vi "Control_HMI.vi"   [LabVIEW 2018]
uses:
  Global/TimerReferences.vi
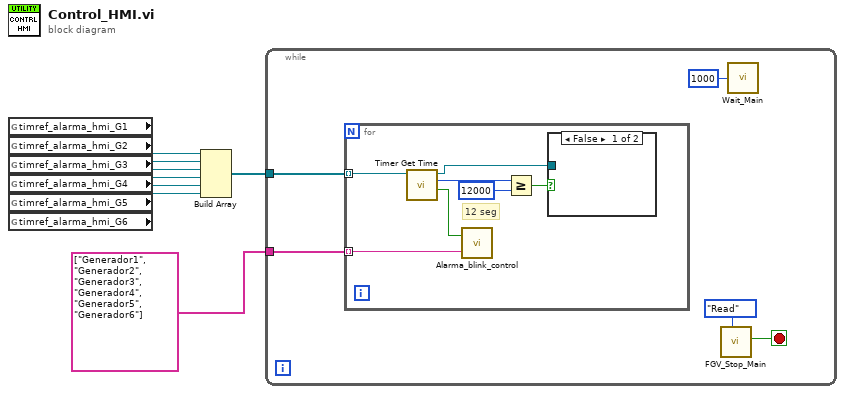
[diagram p0: block diagram]
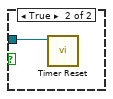
[diagram p2: hidden frame]
diagram:
  n1 = global read "TimerReferences.vi" "timref_alarma_hmi_G1"() -> (w8:refnum<data-value>)
  n2 = global read "TimerReferences.vi" "timref_alarma_hmi_G2"() -> (w7:refnum<data-value>)
  n3 = global read "TimerReferences.vi" "timref_alarma_hmi_G3"() -> (w6:refnum<data-value>)
  n4 = global read "TimerReferences.vi" "timref_alarma_hmi_G4"() -> (w5:refnum<data-value>)
  n5 = global read "TimerReferences.vi" "timref_alarma_hmi_G5"() -> (w4:refnum<data-value>)
  n6 = global read "TimerReferences.vi" "timref_alarma_hmi_G6"() -> (w3:refnum<data-value>)
  n7 = Build Array(w8, w7, w6, w5, w4, w3) -> (w2:refnum<data-value>[])
  n8 = while {
    tunnel: w2 -> [w10]
    tunnel: string[] ["Generador1", "Generador2", "Generador3", "Generador4", "Generador5", "Generador6"] -> [w9]
    stop <- w13 stop-if-true
    n9 = for {
      tunnel: w10 -> [w20] mode=indexing
      tunnel: w9 -> [w16] mode=indexing
      # "12 seg"
      n10 = call "Timer Get Time.vi"("Timer reference"=w20) -> ("Running ?"=w17:bool, "Elapsed Time (ms)"=w19:u32, "Timer reference  out"=w15:refnum<data-value>)  [unwired: 7 in, 1 out]
      n11 = call "Alarma_blink_control.vi"("Nombre"=w16, "alarm"=w17) -> ()  [unwired: 1 in]
      n12 = Greater Or Equal?(x=w19, y=u32 12000) -> (x >= y?=w14:bool)
      n13 = case shown="False" w14 {
        tunnel: w15 -> [_ w21]
        frame False {
        }
        frame True {
          n14 = call "Timer Reset.vi"("Timer reference"=w21) -> ()  [unwired: 9 in, 2 out]
        }
      }
    }
    n15 = call "FGV_Stop_Main.vi"("Action"=enum16{"Read", "Write"}."Read") -> ("Var Out"=w13:bool)  [unwired: 9 in, 1 out]
    n16 = call "Wait_Main.vi"("Wait time (msec)"=u32 1000) -> ()  [unwired: 5 in]
  }
